vi "MyGlobal.vi"() -> ()   [LabVIEW 2011]
panel:
  in  "PWM Scaler":dbl
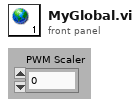
[diagram p1: front panel]
diagram:
